vi "FT10_Semi-Auto Set Power.vi"(7 "Wait Time (ms)":i32=10, 8 "Power Level":T4, 9 "Mode in":T2, 10 "Port in":T3) -> (1 "Mode out":T2, 2 "Port out":T3, 3 "output cluster":T1)   [LabVIEW 2024]
doc: "Creates message for Message Handling Loop to set power level on a specified port & mode."
uses:
  Controls/Control_Semi-Auto Port.ctl
  Controls/Control_Semi-Auto Mode.ctl
  Controls/Control_Semi-Auto Power Level.ctl
  Controls/Control_Command Cluster.ctl
  Controls/Control_Auto Set Power Cluster.ctl
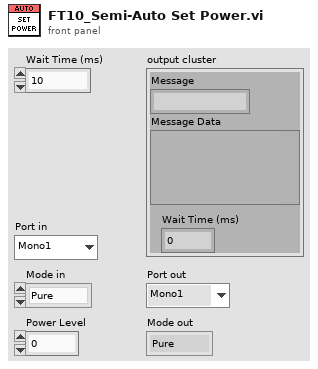
[diagram p1: front panel]
types:
  T1 = typedef "Control_Command Cluster.ctl" = cluster{"Message":string, "Message Data":variant, "Wait Time (ms)":i32}
  T2 = typedef "Control_Semi-Auto Mode.ctl" = enum16{"Pure", "Blend", "Spray", "Fulgerate", "Standard", "Macro", "Precision", "Ligasure", "Error"}
  T3 = typedef "Control_Semi-Auto Port.ctl" = enum16{"Mono1", "Mono2", "Bipolar", "Ligasure", "Error"}
  T4 = typedef "Control_Semi-Auto Power Level.ctl" = dbl
  T5 = typedef "Control_Auto Set Power Cluster.ctl" = cluster{"Port":T3, "Mode":T2, "Power Level":T4}
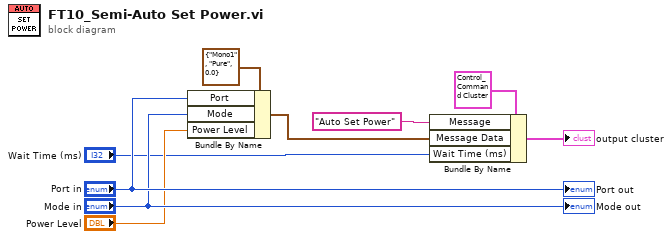
[diagram p0: block diagram]
diagram:
  n1 = Bundle By Name(cluster=T5 {"Port"=enum."Mono1", "Mode"=enum."Pure", "Power Level"=0.0}, "Port"="Port in", "Mode"="Mode in", "Power Level"="Power Level") -> (w4:T5)
  n2 = Bundle By Name(cluster=T1 {"Message"="", "Message Data"=variant, "Wait Time (ms)"=0}, "Message"="Auto Set Power", "Message Data"=w4, "Wait Time (ms)"="Wait Time (ms)") -> (→"output cluster":T1)
  "Port out" <- "Port in"
  "Mode out" <- "Mode in"
